vi "Calbration Engine.vi"(0 "Calibration Actor in":refnum<class "Calibration Actor.lvclass">) -> ()   [LabVIEW 2014, in "Calibration.lvlib" / "Calibration Actor.lvclass"]
doc: "This is the main engine for the calibration configuration. This method will run through the sequence that has been loaded in Pre Init Launch from the appropriate calibration file. The engine will essentially send messages to the controller to initiate commands. There is no waiting for a response."
uses:
  Calibration Actor.lvclass
  SuperActor/SuperActor.lvclass/SuperActor.ctl
  <vilib>/ActorFramework/Actor/Actor.lvclass/Actor.ctl
  <vilib>/ActorFramework/Message Enqueuer/Message Enqueuer.lvclass/Message Enqueuer.ctl
  Calibration Actor.lvclass/Calibration Actor.ctl
  SuperActor/Read Log Session.vi
  <vilib>/ActorFramework/Message Enqueuer/Init from Existing Queue.vi
  <vilib>/ActorFramework/Message Enqueuer/Enqueue.vi
  <vilib>/ActorFramework/Message Priority Queue/Priority Enqueue.vi
  <userlib>/_Session Fwk/Session - Root.lvclass
  <vilib>/ActorFramework/Message Enqueuer/Message Enqueuer.lvclass
  <vilib>/ActorFramework/Stop Msg/Stop Msg.lvclass
  reusable/Sequence/SEQ/SEQ.lvclass
  <vilib>/ActorFramework/Actor/Actor.lvclass
  reusable/Session APIs/Session Log/System Log.lvclass
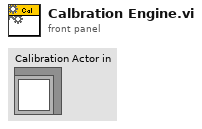
[diagram p1: front panel]
types:
  T1 = typedef "Session - Root.lvclass/Session Handle.ctl" = refnum<data-value>
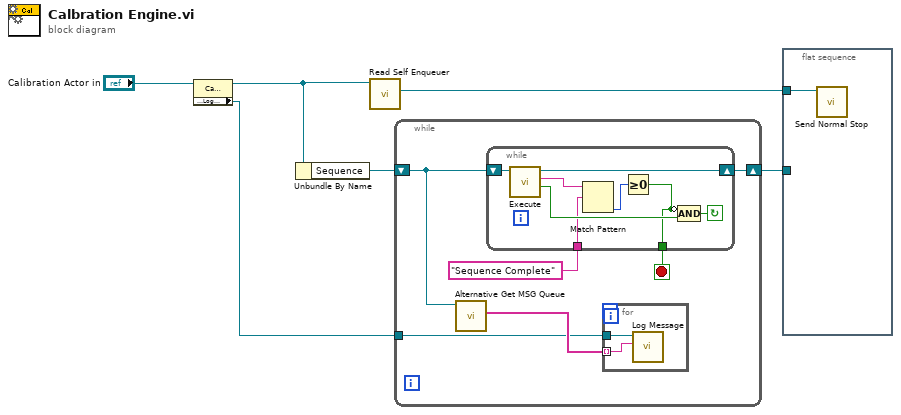
[diagram p0: block diagram]
diagram:
  n1 = property class="Calibration Actor"(reference="Calibration Actor in") -> (reference out=w2:refnum<class "Calibration Actor.lvclass">, "Accessors:Log Session"=w1:T1)  [unwired: 1 in, 1 out]
  n2 = Unbundle By Name(w2) -> ("Sequence"=w6:refnum<class "SEQ.lvclass">)
  n3 = call <vilib>:"Read Self Enqueuer.vi"("Actor"=w2) -> ("Self Enqueuer"=w4:refnum<class "Message Enqueuer.lvclass">)  [unwired: 10 in]
  n4 = while {
    shift-right: [w11] -> w5
    shift-left: w6 -> [w9]
    tunnel: w1 -> [w7]
    stop <- w10 stop-if-true
    n5 = call "Alternative Get MSG Queue.vi"("SEQ in"=w9) -> ("seqMsg"=w8:string[])  [unwired: 9 in, 1 out]
    n6 = while {
      shift-right: [w22] -> w11
      shift-left: w9 -> [w21]
      tunnel: "Sequence Complete" ("y") -> [w18]
      tunnel: [w15] -> w10
      stop <- w19 continue-if-true
      n7 = call-dynamic "Execute.vi"("SEQ in"=w21) -> ("Next Step?"=w20:bool, "MSG"=w17:string, "SEQ out"=w22:refnum<class "SEQ.lvclass">)  [unwired: 7 in, 1 out]
      n8 = Match Pattern(string=w17, regular expression=w18) -> (offset past match=w16:i32)  [unwired: 1 in, 3 out]
      n9 = Greater Or Equal To 0?(x=w16) -> (x >= 0?=w15:bool)
      n10 = Compound Arithmetic op=AND(invert w15, w20) -> (w19:bool)
    }
    n11 = for {
      tunnel: w8 -> [w14] mode=indexing
      tunnel: w7 -> [w13]
      n12 = call "Log Message.vi"("MSG In"=w14, "session in"=w13) -> ()  [unwired: 8 in, 2 out]
    }
  }
  n13 = flat-sequence {
    tunnel: w5 -> [_]
    tunnel: w4 -> [w23]
    frame #0 {
      n14 = call <vilib>:"Send Normal Stop.vi"("Message Enqueuer"=w23) -> ()  [unwired: 10 in, 1 out]
    }
  }
